vi "buildTestScenario.vi"(8 "error in (no error)":errorcluster, 9 "Test Scenario":T1, 10 "Log":refnum<class "ITestLog.lvclass">, 11 "ITestScenarioFactory in":refnum<class "ITestScenarioFactory.lvclass">) -> (0 "error out":errorcluster, 2 "ITestScenario.lvclass":refnum<class "ITestScenario.lvclass">, 3 "ITestScenarioFactory out":refnum<class "ITestScenarioFactory.lvclass">)   [LabVIEW 2015, in "ITestScenarioFactory.lvclass"]
uses:
  ITestScenarioFactory.lvclass
  Typedefs/TestScenarioTypes.ctl
  TestScenario/ITestScenario/ITestScenario.lvclass
  TestLog/ITestLog/ITestLog.lvclass
  Typedefs/ILCBTTypedefs.lvlib
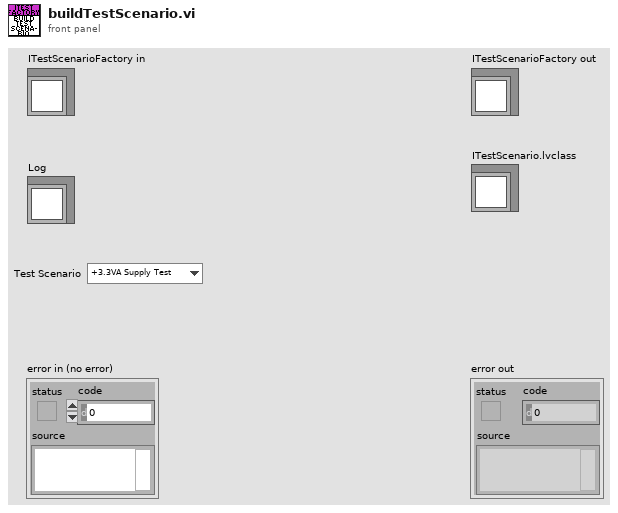
[diagram p1: front panel]
types:
  T1 = typedef "ILCBTTypedefs.lvlib/TestScenarioTypes.ctl" = enum16{"+3.3VA Supply Test", "+3.3VD Supply Test", "+5VA Supply Test", "+5VD Supply Test"}
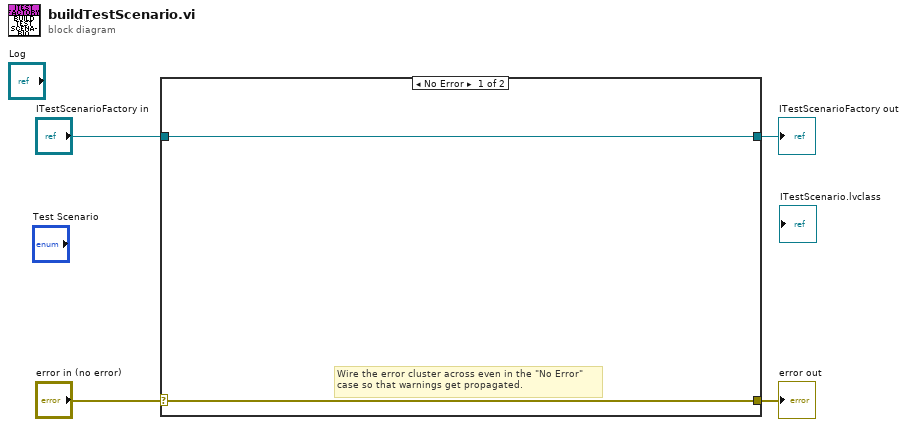
[diagram p0: block diagram]
diagram:
  n1 = case shown="No Error" "error in (no error)" {
    selector: "error in (no error)" -> [w5 w8]
    tunnel: [w5 w8] -> w3
    tunnel: [w6 w7] -> w1
    tunnel: "ITestScenarioFactory in" -> [w6 w7]
    frame No Error {
      # "Wire the error cluster across even in the \"No Error\"\ncase so that warnings get propagated."
    }
    frame Error {
    }
  }
  "error out" <- w3
  "ITestScenarioFactory out" <- w1
